vi "Robot Main.vi"() -> ()   [LabVIEW 2013]
doc: "This VI imlements the framework and scheduler for your robotics program. It should not be necessary to modify the framework. You are expected to add your code to the VIs called from Robot Main, the ones located in the Team Code within the project."
uses:
  <vilib>/Rock Robotics/WPI/Camera/WPI_CameraImageSize.ctl
  2014 Sub VI's/Other/Tellop Shift control.ctl
  2014 Sub VI's/Drive Code/Auto Transmission Code/All Shifter shift register typedef.ctl
  2014 Sub VI's/Drive Code/Auto Transmission Code/Shifter shift typedef.ctl
  2014 Sub VI's/catapult code/catapult shift.ctl
  2014 Sub VI's/catapult code/cataplut states.ctl
  Robot Global Data.vi
  2014 Sub VI's/Robot Global Var.vi
panel:
  in  "Image Size":T1=enum."320x240"
  in  "Enable Vision":bool
  in  "Finish":bool
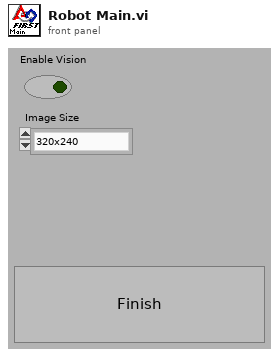
[diagram p1: front panel]
types:
  T1 = typedef "WPI_CameraImageSize.ctl" = enum16{"640x480", "320x240", "160x120"}
  T2 = typedef "Tellop Shift control.ctl" = cluster{"Shifter to Shift":T3, "catapult to shift":T5}
  T3 = typedef "All Shifter shift register typedef.ctl" = cluster{"be in high gear?":bool, "Auto shifter to shift":T4}
  T4 = typedef "Shifter shift typedef.ctl" = u32
  T5 = typedef "catapult shift.ctl" = cluster{" CatapultState":T6, "millisecond timer value in":u32}
  T6 = typedef "cataplut states.ctl" = enum16{"wait for trigger", "firing", "wait for coming back", "wench back"}
  T7 = typedef "Robot dev revs.ctl" = cluster{"Drive":T8, "Catapult devrevs":T29, "Drive Joystick":T32, "Operator Joystick":T32, "roller devrevs":T34, "Puncher devrevs":T35}
  T8 = typedef "Drive typedef.ctl" = cluster{"Drive Actuaters":cluster{"Motor devRevs":T9, "SolenoidDevRef":T18}, "Drive Sensor data":T21}
  T9 = typedef "Drive Motors Typedef.ctl" = cluster{"Left Side Motors":T10, "Right Side Motors":T10, "dev Status":errorcluster}
  T10 = typedef "GearBox Typedef.ctl" = cluster{"Motor 1 devRev":T11, "Motor 2 devRev":T11, "Motor 3 devRev":T11}
  T11 = typedef "WPI_MotorControlDeviceRef.ctl" = cluster{"DeviceStatus":errorcluster, "Type":enum16{"PWM", "CAN"}, "PWM":cluster{"Digital Module":T12, "PWM Channel":T13, "DeadBand":T14}, "CAN":cluster{"Device Number":u8, "Control Mode":T15, "Semaphore":T16, "Max Vout":dbl}, "Invert":bool, "TransformRef":T17, "InvTransformRef":T17}
  T12 = typedef "FPGA_TypedefDigitalModule.ctl" = enum16{"Digital Module 1", "Digital Module 2"}
  T13 = typedef "FPGA_DIOPWMChannel.ctl" = enum8{"PWM 1", "PWM 2", "PWM 3", "PWM 4", "PWM 5", "PWM 6", "PWM 7", "PWM 8", "PWM 9", "PWM 10", "Invalid"}
  T14 = typedef "WPI_PWMDeadband.ctl" = cluster{"Name":string, "maxPositivePwm":i32, "minPositivePwm":i32, "centerPwm":i32, "maxNegativePwm":i32, "minNegativePwm":i32, "angularRange":u16}
  T15 = typedef "WPI_CANJaguar_ControlMode.ctl" = enum8{"Percent VBus", "Current", "Speed", "Position", "Voltage"}
  T16 = typedef "Semaphore RefNum" = refnum<k1>
  T17 = typedef "WPI_PWMTransform_ConPane.ctl" = refnum<vi>
  T18 = typedef "WPI_SolenoidDevRef.ctl" = cluster{"DevStatus":errorcluster, "Solenoid Module":T19, "Forward Solenoid Channel":T20, "Reverse Solenoid Channel":T20}
  T19 = typedef "FPGA_TypedefSolenoidModule.ctl" = enum16{"Solenoid Module 1", "Solenoid Module 2"}
  T20 = typedef "WPI_SolenoidChannel.ctl" = enum8{"Solenoid 1", "Solenoid 2", "Solenoid 3", "Solenoid 4", "Solenoid 5", "Solenoid 6", "Solenoid 7", "Solenoid 8", "Invalid"}
  T21 = typedef "Drive Sensor Typedef.ctl" = cluster{"Encoders":cluster{"Right Encoder":T22}, "GyroDevRef":T26, "Last commanded Angle":dbl}
  T22 = typedef "WPI_EncoderDevRef.ctl" = cluster{"DevStatus":errorcluster, "EncoderIndex":T23, "CounterIndex":T24, "DistancePerCount":dbl, "Decoding Type":T25}
  T23 = typedef "FPGA_EncoderIdx.ctl" = enum8{"Enc 0", "Enc 1", "Enc 2", "Enc 3", "Invalid"}
  T24 = typedef "FPGA_CounterCtrSystemIndex.ctl" = enum8{"Ctr 0", "Ctr 1", "Ctr 2", "Ctr 3", "Ctr 4", "Ctr 5", "Ctr 6", "Ctr 7", "Invalid"}
  T25 = typedef "WPI_EncoderType.ctl" = enum16{"1x", "2x", "4x"}
  T26 = typedef "WPI_GyroDevRef.ctl" = cluster{"DevStatus":errorcluster, "Analog Module":T27, "Analog Channel":T28, "Offset":dbl, "Gain (VoltsPerDegree/Second)":dbl}
  T27 = typedef "FPGA_TypedefAnalogModule.ctl" = enum16{"Analog Module 1", "Analog Module 2"}
  T28 = typedef "FPGA_AIChannel.ctl" = enum8{"AI 1", "AI 2", "AI 3", "AI 4", "AI 5", "AI 6", "AI 7", "AI 8", "Invalid"}
  T29 = typedef "catapult type def.ctl" = cluster{"MotorControlDeviceRef":T11, "SolenoidDevRef":T18, "first limit switch":T30, "second limit switch":T30}
  T30 = typedef "WPI_DigitalInputDevRef.ctl" = cluster{"DevStatus":errorcluster, "DIO Channel":T31, "Digital Module":T12}
  T31 = typedef "FPGA_DIOChannel.ctl" = enum8{"DIO 1", "DIO 2", "DIO 3", "DIO 4", "DIO 5", "DIO 6", "DIO 7", "DIO 8", "DIO 9", "DIO 10", "DIO 11", "DIO 12", "DIO 13", "DIO 14", "Invalid"}
  T32 = typedef "WPI_JoystickDevRef.ctl" = cluster{"Device":T33}
  T33 = typedef "WPI_JoystickDeviceEnum.ctl" = enum16{"USB 1", "USB 2", "USB 3", "USB 4", "Kinect 1", "Kinect 2"}
  T34 = typedef "roller typedef.ctl" = cluster{"SolenoidDevRef":T18, "MotorControlDeviceRef":T11, "DigitalInputDevRef":T30}
  T35 = typedef "Puncher type.ctl" = cluster{"SolenoidDevRef":T18, "DigitalInputDevRef":T30}
  T36 = typedef "WPI_DriverStationMatch Info.ctl" = cluster{"Autonomous Elapsed Seconds":dbl, "TeleOp Elapsed Seconds":dbl, "Disabled Elapsed Seconds":dbl, "Visited Autonomous":bool, "Visited TeleOp":bool, "Visited Disabled":bool, "Autonomous Settings":cluster{"Autonomous Style":enum16{"Iterative", "Independent"}, "VI Refnum":refnum<vi>}}
  T37 = typedef "WPI_DriverStationDerivedRobotMode.ctl" = enum16{"Init", "Execute", "Stop"}
  T38 = typedef "WPI_DriverStationRobotMode2.ctl" = enum16{"Autonomous Disabled", "Autonomous Enabled", "Teleop Disabled", "Teleop Enabled", "Timeout", "Finish", "Test Disabled", "Test Enabled"}
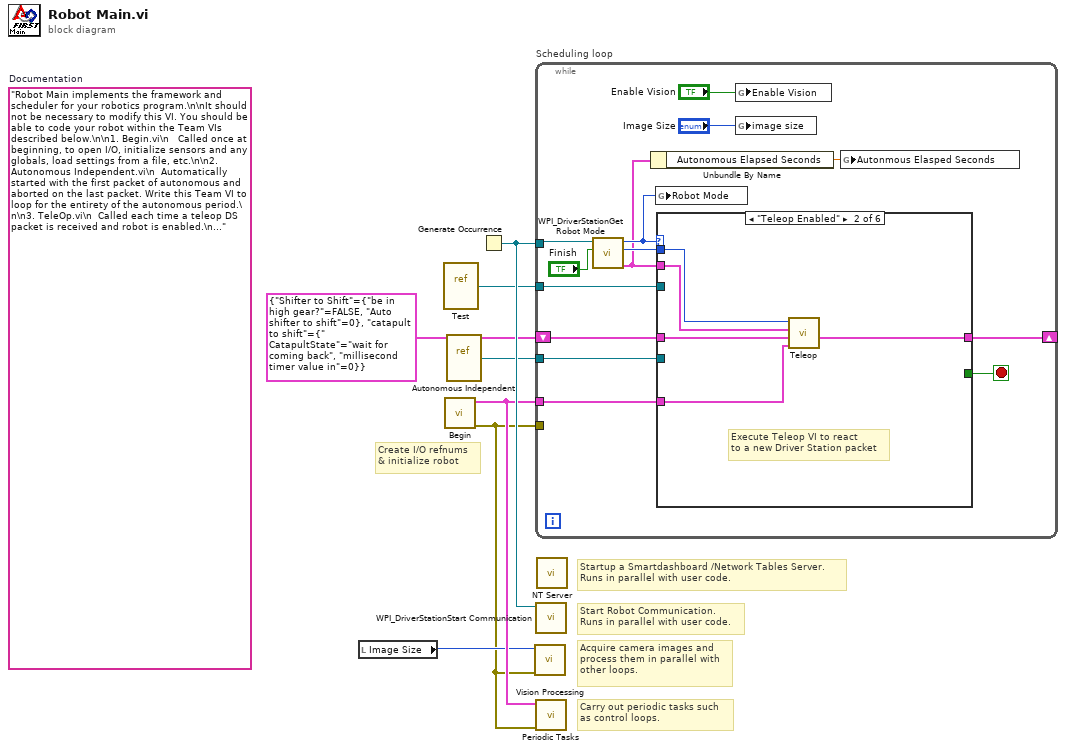
[diagram p0: block diagram]
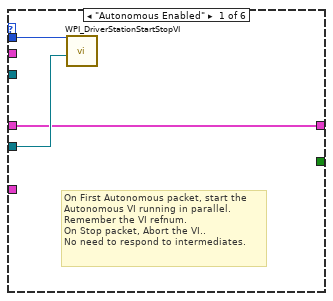
[diagram p2: hidden frame]
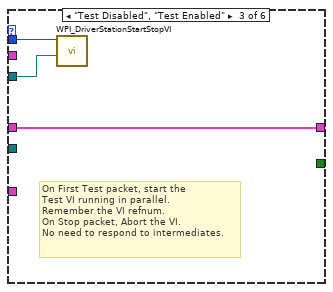
[diagram p3: hidden frame]
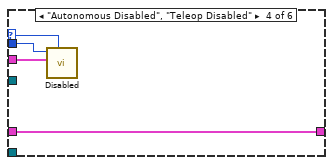
[diagram p4: hidden frame]
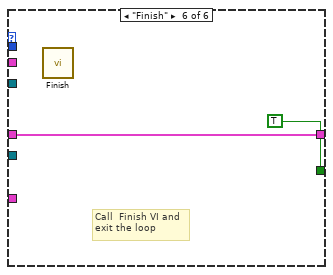
[diagram p6: hidden frame]
diagram:
  (unwired) "Robot Main implements the framework and scheduler for your robotics program.\n\nIt should not be necessary to modify this VI. You should be able to code your robot within the Team VIs described below.\n\n1. Begin.vi\n   Called once at beginning, to open I/O, initialize sensors and any globals, load settings from a file, etc.\n\n2. Autonomous Independent.vi\n  Automatically started with the first packet of autonomous and aborted on the last packet. Write this Team VI to loop for the entirety of the autonomous period.\n\n3. TeleOp.vi\n  Called each time a teleop DS packet is received and robot is enabled.\n\n4. Disabled.vi\n  Called each time a packet is received and the robot is disabled.\n\n5. Test.vi\n  Called Automatically started with the first test packet and aborted on the last. Modify this VI to carry out robot and sensor validation tests.\n\n6. Vision.vi\n  A parallel loop that acquires and processes camera images.\n\n7. PeriodicTasks.vi\n  Parallel loops running at user-defined rates.\n\n8. Finish.vi\n  Called before exiting, so you can save data, clean up I/O, etc.\n"  # Documentation
  # "Startup a Smartdashboard /Network Tables Server.\nRuns in parallel with user code."
  # "Carry out periodic tasks such\nas control loops."
  # "Acquire camera images and\nprocess them in parallel with\nother loops."
  # "Create I/O refnums\n& initialize robot"
  # "Start Robot Communication.\nRuns in parallel with user code."
  n1 = local read "Image Size"() -> (w3:T1)
  n2 = vi-ref "Test.vi"() -> (w5:refnum<vi>)
  n3 = call "Begin.vi"() -> ("error out"=w2:errorcluster, "Robot dev revs"=w4:T7)  [unwired: 1 in, 9 out]
  n4 = vi-ref "Autonomous Independent.vi"() -> (w6:refnum<vi>)
  n5 = Generate Occurrence() -> (w7:refnum<k4>)
  n6 = call "Vision Processing.vi"("error in (no error)"=w2, "Image Size"=w3) -> ()  [unwired: 6 in]
  n7 = while "Scheduling loop" {
    tunnel: w7 -> [w20]
    tunnel: w2 -> [_]
    tunnel: w6 -> [w16]
    tunnel: w5 -> [w14]
    shift-right: [w12] -> _
    shift-left: T2 {"Shifter to Shift"={"be in high gear?"=FALSE, "Auto shifter to shift"=0}, "catapult to shift"={" CatapultState"=enum."wait for coming back", "millisecond timer value in"=0}} ("Tellop to shift") -> [w11]
    tunnel: w4 -> [w10]
    stop <- w18 stop-if-true
    n8 = call <vilib>:"WPI_DriverStationGet Robot Mode.vi"("Finish"="Finish", "DS Occurrence"=w20) -> ("Match Info out"=w9:T36, "Call Context"=w21:T37, "Robot Mode"=w13:T38)  [unwired: 7 out]
    n9 = Unbundle By Name(w9) -> ("Autonomous Elapsed Seconds"=w8:dbl)
    n10 = global write "Robot Global Data.vi" "Robot Mode"(w13) -> ()
    n11 = case shown="\"Teleop Enabled\"" w13 {
      selector: w13 -> [_ _ _ w34 _ _]
      tunnel: w21 -> [w24 w29 w32 w36 _ _]
      tunnel: w9 -> [_ w28 _ w35 _ _]
      tunnel: [_ _ _ _ _ TRUE] -> w18
      tunnel: w16 -> [w23 _ _ _ _ _]
      tunnel: w14 -> [_ _ w31 _ _ _]
      tunnel: [w22 w27 w30 w33 w37 w38] -> w12
      tunnel: w11 -> [w22 w26 w30 w33 w37 w38]
      tunnel: w10 -> [_ w25 _ _ _ _]
      frame "Autonomous Enabled" {
        # "On First Autonomous packet, start the\nAutonomous VI running in parallel.\nRemember the VI refnum.\nOn Stop packet, Abort the VI..\nNo need to respond to intermediates."
        n12 = call <vilib>:"WPI_DriverStationStartStopVI.vi"("VI in"=w23, "Call Context"=w24) -> ()  [unwired: 10 in]
      }
      frame "Teleop Enabled" {
        # "Execute Teleop VI to react\nto a new Driver Station packet"
        n13 = call "Teleop.vi"("Robot dev revs"=w25, "Tellop from shift"=w26, "Match Info"=w28, "Call Context"=w29) -> ("Tellop to shift"=w27:T2)  [unwired: 7 out]
      }
      frame "Test Disabled", "Test Enabled" {
        # "On First Test packet, start the\nTest VI running in parallel.\nRemember the VI refnum.\nOn Stop packet, Abort the VI.\nNo need to respond to intermediates."
        n14 = call <vilib>:"WPI_DriverStationStartStopVI.vi"("VI in"=w31, "Call Context"=w32) -> ()  [unwired: 10 in]
      }
      frame "Autonomous Disabled", "Teleop Disabled" {
        n15 = call "Disabled.vi"("Robot Mode"=w34, "Match Info"=w35, "Call Context"=w36) -> ()  [unwired: 2 in, 7 out]
      }
      frame "Timeout" {
        # "Driver Station packet didn't arrive.\nPossibly useful for diagnostics"
      }
      frame "Finish" {
        # "Call  Finish VI and\nexit the loop"
        n16 = call "Finish.vi"() -> ()  [unwired: 1 in, 7 out]
      }
    }
    n17 = global write "Robot Global Data.vi" "Enable Vision"("Enable Vision") -> ()
    n18 = global write "Robot Global Data.vi" "image size"("Image Size") -> ()
    n19 = global write "Robot Global Var.vi" "Autonmous Elasped Seconds"(w8) -> ()
  }
  n20 = call <vilib>:"WPI_DriverStationStart Communication.vi"("occurrence"=w7) -> ()  [unwired: 11 out]
  n21 = call "Periodic Tasks.vi"("error in"=w2, "Robot dev revs"=w4) -> ()  [unwired: 10 out]
  n22 = call <vilib>:"NT Server.vi"() -> ()  [unwired: 12 in]
